vi "pix2um&refsubstract.vi"(3 "ref substract":bool, 4 "XYZ in":dbl[][][](array[numeric])) -> (1 "xyz um out":dbl[][][](array[numeric]))   [LabVIEW 2011, in "OfflineTracker.lvlib"]
uses:
  OfflineTracker.lvlib
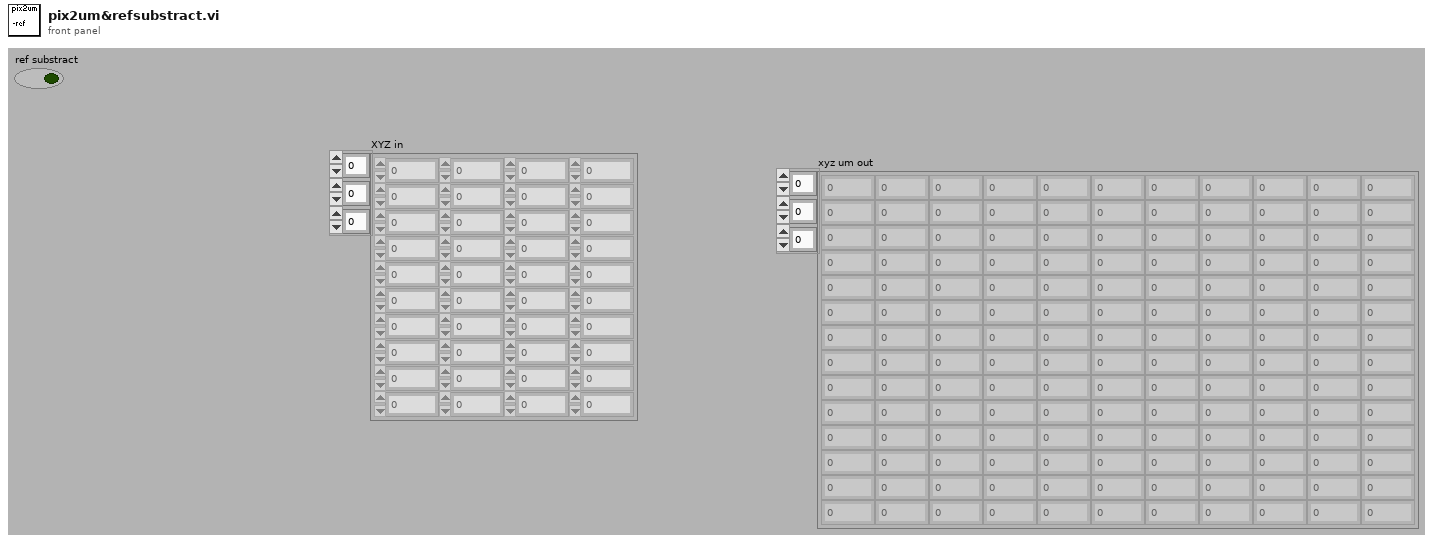
[diagram p1: front panel]
types:
  T1 = typedef "IMAQ Image.ctl" = refnum<image>
  T2 = cluster{"front panel settings":cluster{"files":cluster{"LUT path":path, "Trace path":path, " folders #":i32, "base path":path, "use trace":bool, "use base":bool, "LUT tmp":i32, "Trace tmp":i32, "active path":path}, "Tracking":cluster{"RminZ (pix)":i32, "Rmax (pix)":i32, "angular pixel \ncoverage factor":dbl, "radial pixel \ncoverage factor":dbl}, "Frames":cluster{"Start frame":i32, "number of frames":u32, "display frame ":i32, "track every nd frame ":i32, "Track all frames":bool, "active frame":i32}, "Calibs":cluster{"Zlut number of steps":i32, "pix/um":dbl, "Z correction factor":dbl, "Zlut step size (um)":dbl, "ROI(pix)":i32}, "Beads":cluster{"number of ref beads":i32, "overlay":bool}, "Misc":cluster{"save images to new location":bool, "destination":path}}, "data":cluster{"Image":T1, "image size":i32[], "Bead Array":i32[][], "overlay image":T1, "# beads":i32, "Job list":string[][], "job running":bool, "job #":i32, "folders to go":i32}}
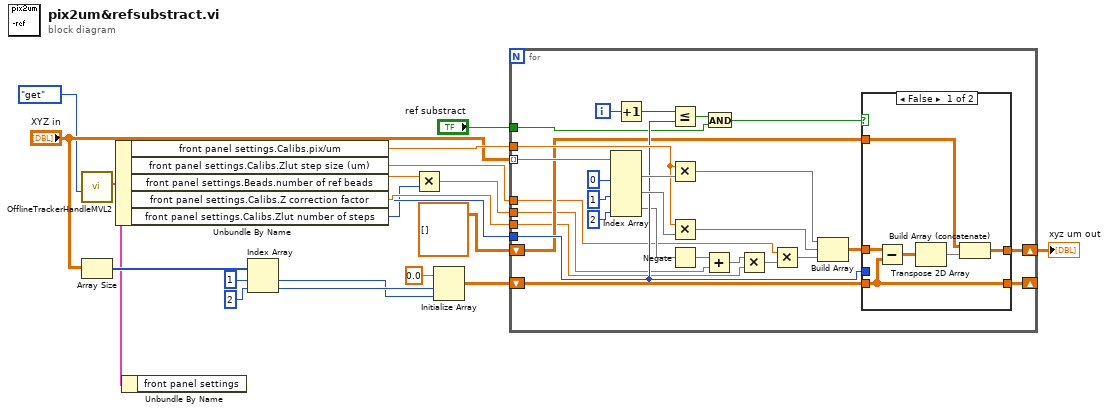
[diagram p0: block diagram]
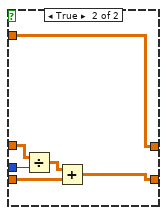
[diagram p2: hidden frame]
diagram:
  n1 = call "OfflineTrackerHandleMVL2.vi"("action"=enum16{"get", "set"}."get") -> ("out"=w1:T2)  [unwired: 5 in, 1 out]
  n2 = Array Size(array="XYZ in") -> (size(s)=w12:i32[])
  n3 = Unbundle By Name(w1) -> ("front panel settings.Calibs.pix/um"=w17:dbl, "front panel settings.Calibs.Zlut step size (um)"=w5:dbl, "front panel settings.Beads.number of ref beads"=w15:i32, "front panel settings.Calibs.Z correction factor"=w18:dbl, "front panel settings.Calibs.Zlut number of steps"=w4:i32)
  n4 = Unbundle By Name(w1) -> ()  [unwired: 1 out]
  n5 = Index Array(array=w12, index #1=1 ("index"), index #2=2 ("index")) -> (element #1=w6:i32, element #2=w7:i32)
  n6 = Multiply(x=w5, y=w4) -> (x*y=w3:dbl)
  n7 = Initialize Array(0.0 ("element"), w7, w6) -> (w8:dbl[][])
  n8 = for {
    tunnel: "XYZ in" -> [w47] mode=indexing
    tunnel: w17 -> [w41]
    tunnel: w18 -> [w21]
    tunnel: w5 -> [w20]
    shift-right: [w30] -> w19
    shift-left: dbl[][][] [] -> [w29]
    tunnel: w15 -> [w33]
    shift-right: [w32] -> _
    shift-left: w8 -> [w31]
    tunnel: "ref substract" -> [w26]
    tunnel: w3 -> [w23]
    i -> [w36]
    n9 = Index Array(array=w47, index (col) #1=0 ("disabled index (col)"), index (col) #2=1 ("index (col)"), index (col) #3=2 ("index (col)")) -> (element #1=w43:dbl[], element #2=w42:dbl[], element #3=w25:dbl[])  [unwired: 3 in]
    n10 = Increment(x=w36) -> (x+1=w35:i32)
    n11 = Less Or Equal?(x=w35, y=w33) -> (x <= y?=w28:bool)
    n12 = Multiply(x=w41, y=w43) -> (x*y=w39:dbl[])
    n13 = Multiply(x=w41, y=w42) -> (x*y=w38:dbl[])
    n14 = Negate(x=w25) -> (-x=w24:dbl[])
    n15 = Add(x=w24, y=w23) -> (x+y=w22:dbl[])
    n16 = And(x=w28, y=w26) -> (x .and. y?=w27:bool)
    n17 = Multiply(x=w22, y=w21) -> (x*y=w40:dbl[])
    n18 = Multiply(x=w20, y=w40) -> (x*y=w37:dbl[])
    n19 = Build Array(w39, w38, w37) -> (w34:dbl[][])
    n20 = case shown="False" w27 {
      tunnel: w31 -> [w48 w54]
      tunnel: w34 -> [w50 w59]
      tunnel: w33 -> [_ w58]
      tunnel: [w48 w56] -> w32
      tunnel: [w53 w55] -> w30
      tunnel: w29 -> [w52 w55]
      frame False {
        n21 = Subtract(x=w50, y=w48) -> (x-y=w49:dbl[][])
        n22 = Transpose 2D Array(2D array=w49) -> (transposed array=w51:dbl[][])
        n23 = Build Array (concatenate)(w52, w51) -> (w53:dbl[][][])
      }
      frame True {
        n24 = Divide(x=w59, y=w58) -> (x/y=w57:dbl[][])
        n25 = Add(x=w57, y=w54) -> (x+y=w56:dbl[][])
      }
    }
  }
  "xyz um out" <- w19
